vi "Replace FL Channels.vi"(8 "error in (no error)":errorcluster, 11 "Performanced XNET CAN Signal Logger in":refnum<class "Performanced XNET CAN Signal Logger.lvclass">) -> (0 "error out":errorcluster, 3 "Performanced XNET CAN Signal Logger out":refnum<class "Performanced XNET CAN Signal Logger.lvclass">)   [LabVIEW 2021, in "Performanced XNET CAN Signal Logger.lvlib" / "Performanced XNET CAN Signal Logger.lvclass"]
uses:
  Performanced XNET CAN Signal Logger.lvclass
  <vilib>/FlexLogger/SDK/PluginSDK.lvlibp/PEFClasses/SDK/Producer Channel/Create Producer Channel.vi
  <vilib>/FlexLogger/SDK/PluginSDK.lvlibp/PEFClasses/SDK/Plugin/Plugin.lvclass
  <vilib>/FlexLogger/SDK/PluginSDK.lvlibp
  <vilib>/FlexLogger/SDK/PluginSDK.lvlibp/PEFClasses/SDK/Producer Channel/Producer Channel.lvclass
  C:/Program Files/National Instruments/LabVIEW 2021/vi.lib/FlexLogger/SDK/PluginSDK.lvlibp/PEFClasses/SDK/Plugin/Plugin.lvclass
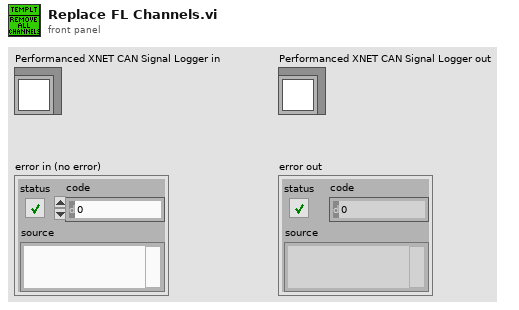
[diagram p1: front panel]
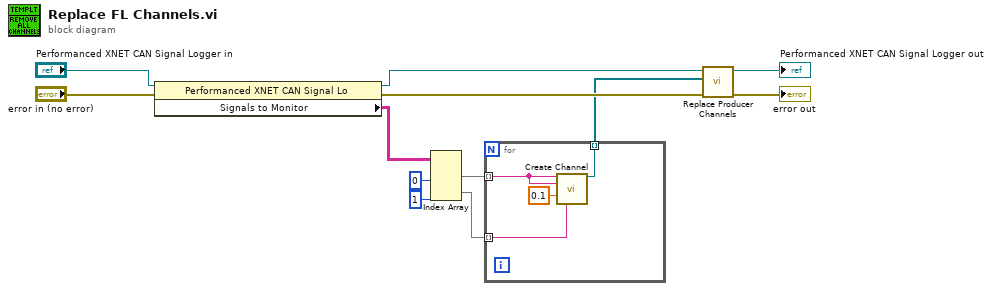
[diagram p0: block diagram]
diagram:
  n1 = property class="Performanced XNET CAN Signal Lo"(reference="Performanced XNET CAN Signal Logger in", error in="error in (no error)") -> (reference out=w12:refnum<class "Performanced XNET CAN Signal Logger.lvclass">, error out=w8:errorcluster, "Signals to Monitor"=w6:string[][])
  n2 = Index Array(array=w6, index (col) #1=0 ("disabled index (col)"), index (col) #2=1 ("index (col)")) -> (element #1=w3:string[], element #2=w2:string[])  [unwired: 2 in]
  n3 = for {
    tunnel: w3 -> [w15] mode=indexing
    tunnel: w2 -> [w16] mode=indexing
    tunnel: [w14] -> w1 mode=indexing
    n4 = call-poly <vilib>:"Create Channel.vi"("Unique Channel Identifier"=w15, "Default Channel Name"=w15, "dt(sec)"=0.1, "Unit"=w16) -> ("Producer Channel"=w14:refnum<class "Producer Channel.lvclass">)  [unwired: 10 in, 1 out]
  }
  n5 = call <vilib>:"Replace Producer Channels.vi"("error in (no error)"=w8, "Producer Channels"=w1, "Plugin"=w12) -> ("error out"=→"error out":errorcluster, "Plugin"=→"Performanced XNET CAN Signal Logger out":refnum<class "Performanced XNET CAN Signal Logger.lvclass">)  [unwired: 7 in]
